vi "Get Next Test.vi"(8 "error in (no error)":errorcluster, 9 "Active Unique ID":string, 11 "ITest Executive in":refnum<class "ITest Executive.lvclass">) -> (0 "error out":errorcluster, 1 "Active Unique ID out":string, 2 "Test":refnum<class "Executioner.lvclass">, 3 "ITest Executive out":refnum<class "ITest Executive.lvclass">, 4 "Found":bool, 5 "Test Executive Ref out":refnum<data-value>, 6 "Complete":bool)   [LabVIEW 2019, in "Test Executive.lvlib" / "ITest Executive.lvclass"]
uses:
  <vilib>/gpm_packages/@cs/test-executive/Source/Test Executive/ITestExecutive/ITest Executive.lvclass
  <vilib>/gpm_packages/@cs/test-executive/Source/Test Executive/Executioner/Executioner.lvclass
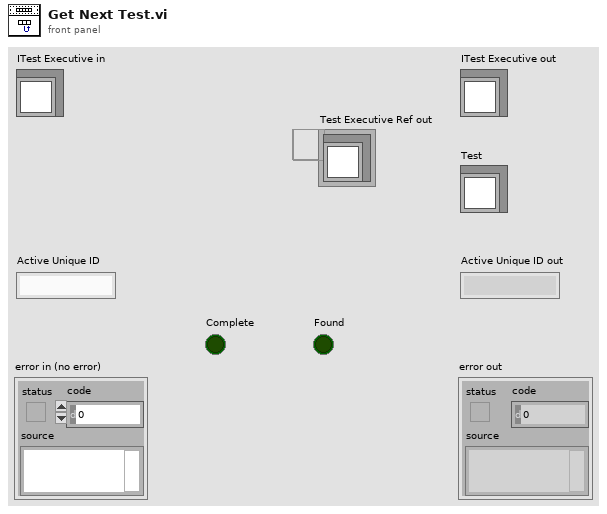
[diagram p1: front panel]
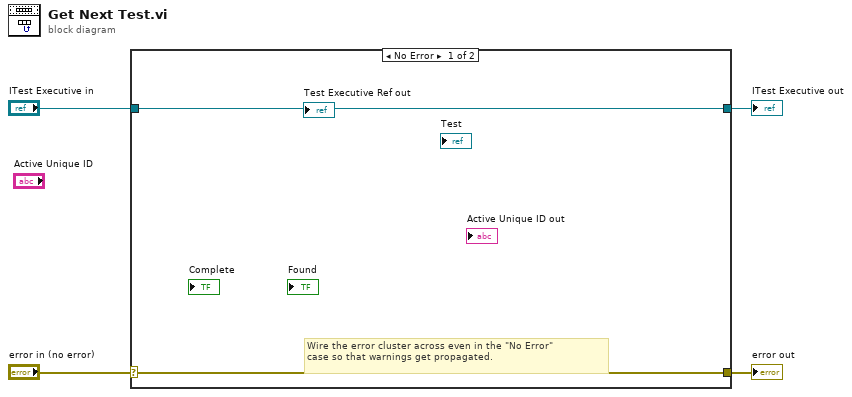
[diagram p0: block diagram]
diagram:
  n1 = case shown="No Error" "error in (no error)" {
    selector: "error in (no error)" -> [w5 w8]
    tunnel: [w5 w8] -> w3
    tunnel: [w6 w7] -> w1
    tunnel: "ITest Executive in" -> [w6 w7]
    frame No Error {
      # "Wire the error cluster across even in the \"No Error\"\ncase so that warnings get propagated."
    }
    frame Error {
    }
  }
  "error out" <- w3
  "ITest Executive out" <- w1
